vi "SMU Testbench.vi"() -> (15 "error out":errorcluster)   [LabVIEW 2018]
uses:
  <instrlib>/niDCPower/nidcpower.llb/niDCPower Source Mode.ctl
  <instrlib>/niDCPower/nidcpower.llb/niDCPower Output Function.ctl
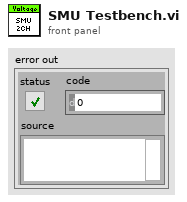
[diagram p1: front panel]
types:
  T1 = typedef "niDCPower Output Function.ctl" = i32
  T2 = typedef "niDCPower Source Mode.ctl" = i32
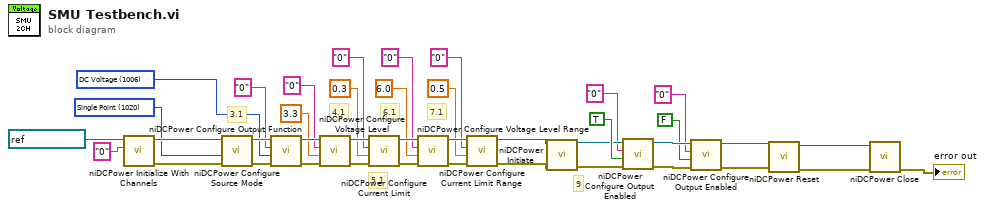
[diagram p0: block diagram]
diagram:
  w19 = T1 1006 items=["DC Voltage"=1006, "DC Current"=1007, "Pulse Voltage"=1049, "Pulse Current"=1050] ("output function")
  w21 = T2 1020 items=["Single Point"=1020, "Sequence"=1021] ("source mode")
  # "7.1"
  # "6.1"
  # "3.1"
  # "5.1"
  # "4.1"
  # "9"
  n1 = call <instrlib>:"niDCPower Initialize With Channels.vi"("channels"="0", "resource name"=refnum<k15> "PXI1Slot2") -> ("error out"=w26:errorcluster, "instrument handle out"=w27:refnum<k15>)  [unwired: 8 in]
  n2 = call <instrlib>:"niDCPower Configure Source Mode.vi"("error in (no error)"=w26, "source mode"=w21, "instrument handle"=w27) -> ("error out"=w25:errorcluster, "instrument handle out"=w24:refnum<k15>)  [unwired: 7 out]
  n3 = call <instrlib>:"niDCPower Configure Output Function.vi"("error in (no error)"=w25, "output function"=w19, "channel name"="0", "instrument handle"=w24) -> ("error out"=w40:errorcluster, "instrument handle out"=w39:refnum<k15>)  [unwired: 6 out]
  n4 = call <instrlib>:"niDCPower Configure Voltage Level.vi"("error in (no error)"=w40, "voltage level"=3.3, "channel name"="0", "instrument handle"=w39) -> ("error out"=w34:errorcluster, "instrument handle out"=w33:refnum<k15>)  [unwired: 6 out]
  n5 = call <instrlib>:"niDCPower Configure Current Limit.vi"("error in (no error)"=w34, "current limit"=0.3, "channel name"="0", "instrument handle"=w33) -> ("error out"=w35:errorcluster, "instrument handle out"=w36:refnum<k15>)  [unwired: 1 in, 5 out]
  n6 = call <instrlib>:"niDCPower Configure Voltage Level Range.vi"("error in (no error)"=w35, "voltage level range"=6.0, "channel name"="0", "instrument handle"=w36) -> ("error out"=w37:errorcluster, "instrument handle out"=w38:refnum<k15>)  [unwired: 6 out]
  n7 = call <instrlib>:"niDCPower Configure Current Limit Range.vi"("error in (no error)"=w37, "current limit range"=0.5, "channel name"="0", "instrument handle"=w38) -> ("error out"=w28:errorcluster, "instrument handle out"=w29:refnum<k15>)  [unwired: 6 out]
  n8 = call <instrlib>:"niDCPower Initiate.vi"("error in (no error)"=w28, "instrument handle"=w29) -> ("error out"=w30:errorcluster, "instrument handle out"=w31:refnum<k15>)  [unwired: 2 in, 6 out]
  n9 = call <instrlib>:"niDCPower Configure Output Enabled.vi"("error in (no error)"=w30, "output enabled"=TRUE, "channel name"="0", "instrument handle"=w31) -> ("error out"=w9:errorcluster, "instrument handle out"=w10:refnum<k15>)  [unwired: 6 in]
  n10 = call <instrlib>:"niDCPower Configure Output Enabled.vi"("error in (no error)"=w9, "output enabled"=FALSE, "channel name"="0", "instrument handle"=w10) -> ("error out"=w3:errorcluster, "instrument handle out"=w4:refnum<k15>)  [unwired: 6 in]
  n11 = call <instrlib>:"niDCPower Reset.vi"("error in (no error)"=w3, "instrument handle"=w4) -> ("error out"=w1:errorcluster, "instrument handle out"=w2:refnum<k15>)  [unwired: 8 in]
  n12 = call <instrlib>:"niDCPower Close.vi"("error in (no error)"=w1, "instrument handle"=w2) -> ("error out"=→"error out":errorcluster)  [unwired: 9 in]
